vi "MeasInductance.vi"() -> ()   [LabVIEW 2017]
uses:
  <vilib>/Analysis/6fits.llb/Curve Fitting Criteria.ctl
  <vilib>/Analysis/NI_AALPro.lvlib
  Keysight N8731A conversion/Keysight N8900 Series.lvlib
panel:
  in  "filename":string caption="Discard data if empty"
  out "Resistance":dbl
  out "Inductance":dbl
  out "V(I)":T1(graph)
  out "Time Data":dbl[](array[numeric])
  out "Voltage Data":dbl[](array[numeric])
  out "Current Data":dbl[](array[numeric])
  out "I(t)":T1(graph)
  in  "stop":bool
  out "start time":dbl format="%_19f"
  in  "Measurement time [s]":dbl=240.0
  in  "OV Value (10V)":dbl=10.0
  in  "VISA resource name":refnum<visa-resource-name>
  in  "Keithley (1)/PSU (0)":bool=TRUE caption="Voltage Source"
  in  "Voltage limit [V]":dbl
  in  "Current limit [A]":dbl
  in  "Time between measurements [ms]":dbl
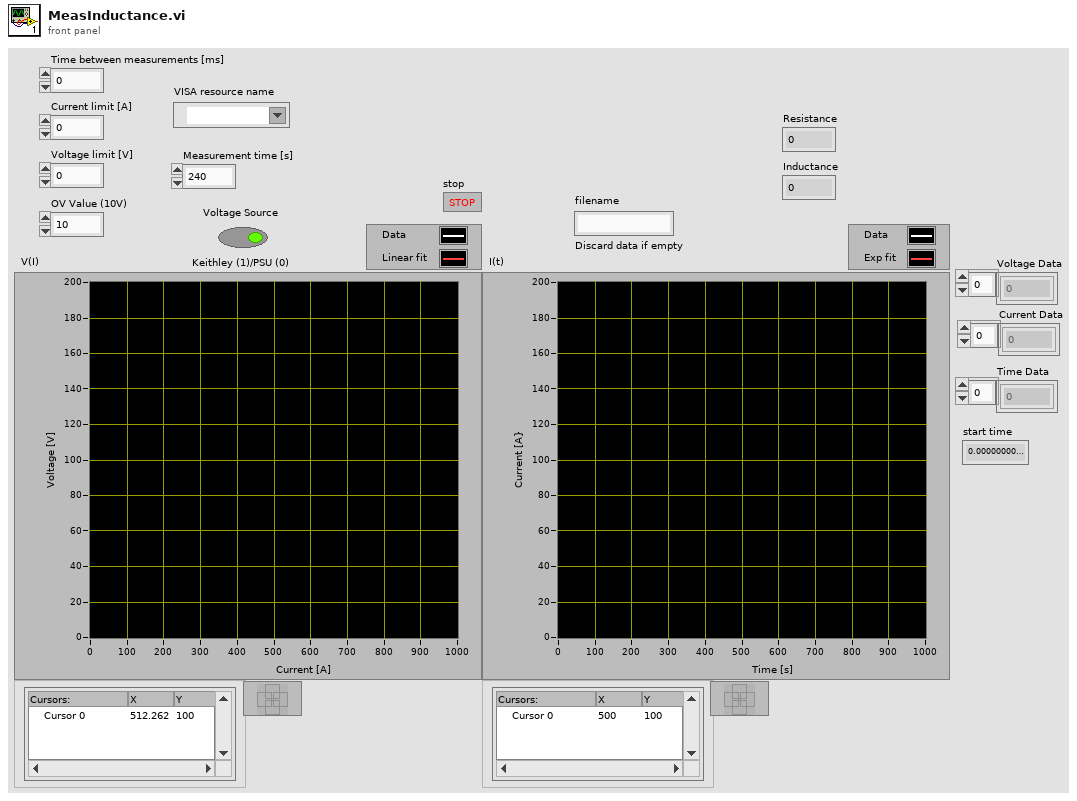
[diagram p1: front panel]
types:
  T1 = cluster{"Current Data":dbl[], "Best Linear Fit":dbl[]}[]
  T2 = cluster{"amp min":dbl, "amp max":dbl, "damping min":dbl, "damping max":dbl, "offset min":dbl, "offset max":dbl}
  T3 = typedef "NI_AALPro.lvlib/Curve Fitting Criteria.ctl" = u16
  T4 = cluster{"Current Data":dbl[], "Best Linear Fit":dbl[]}
  T5 = cluster{"Current Data":dbl[], "Voltage Data":dbl[]}
  T6 = cluster{"Time Data":dbl[], "Best Exponential Fit":dbl[]}
  T7 = cluster{"Time Data":dbl[], "Best Exponential Fit":dbl[]}[]
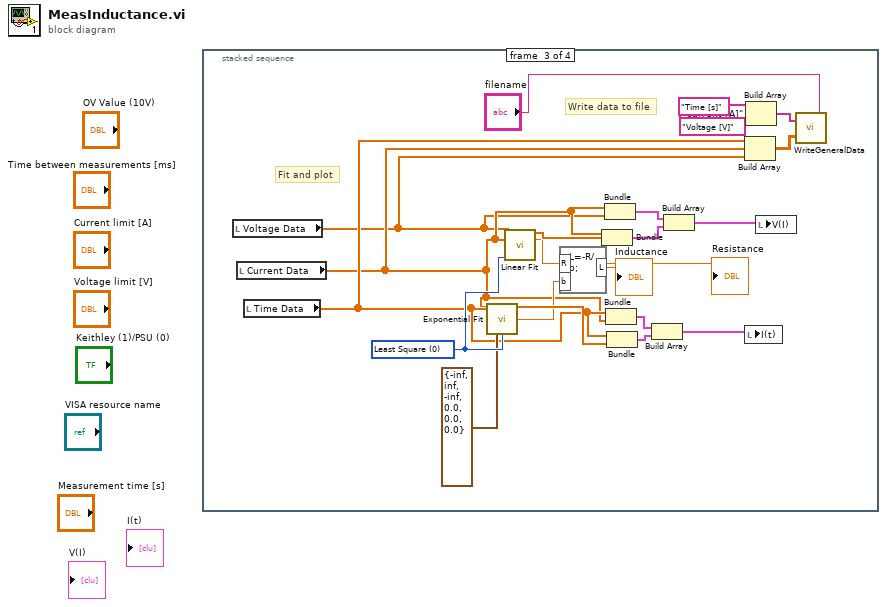
[diagram p0: block diagram]
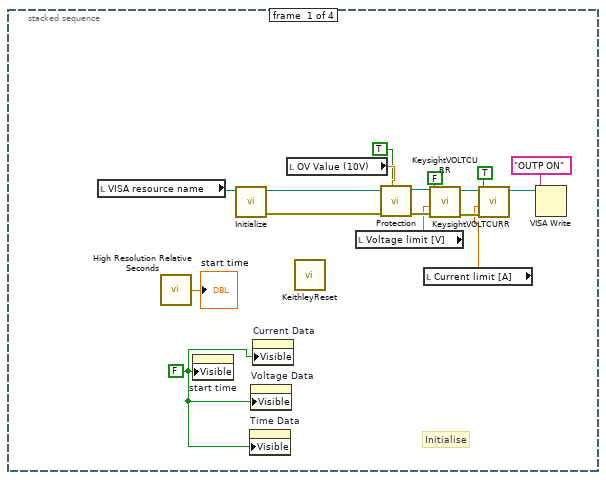
[diagram p2: hidden frame]
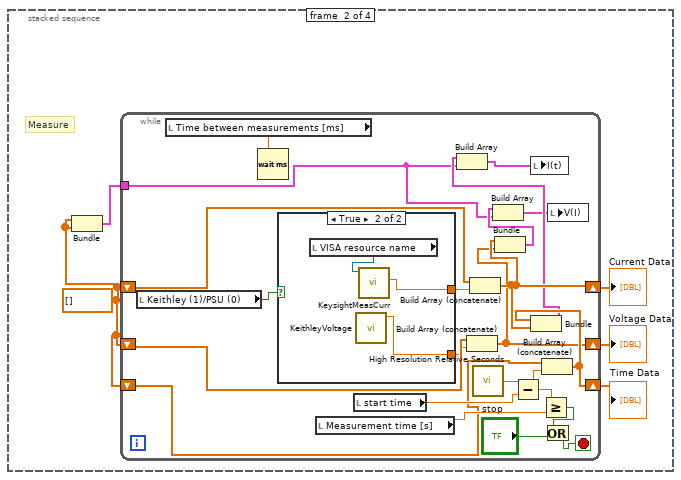
[diagram p3: hidden frame]
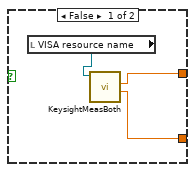
[diagram p4: hidden frame]
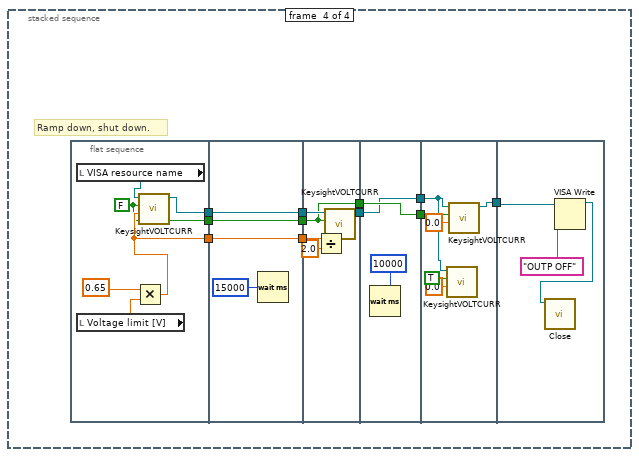
[diagram p5: hidden frame]
diagram:
  n1 = stacked-sequence {
    frame #0 {
      w3 = FALSE ("Visible")
      # "Initialise"
      n2 = local read "VISA resource name"() -> (w15:refnum<visa-resource-name>)
      n3 = call <vilib>:"High Resolution Relative Seconds.vi"() -> ("relative seconds"=→"start time":dbl)
      n4 = property on="start time" class="DigNum (strict)"("Visible"=w3) -> ()  [unwired: 2 in, 2 out]
      n5 = call "Initialize.vi"("VISA resource name"=w15) -> ("error out"=w17:errorcluster, "VISA resource name out"=w16:refnum<visa-resource-name>)  [unwired: 9 in]
      n6 = property on="Time Data" class="Arr (strict)"("Visible"=w3) -> ()  [unwired: 2 in, 2 out]
      n7 = property on="Voltage Data" class="Arr (strict)"("Visible"=w3) -> ()  [unwired: 2 in, 2 out]
      n8 = property on="Current Data" class="Arr (strict)"("Visible"=w3) -> ()  [unwired: 2 in, 2 out]
      n9 = local read "OV Value (10V)"() -> (w14:dbl)
      n10 = call "KeithleyReset.vi"() -> ()  [unwired: 11 in, 1 out]
      n11 = local read "Voltage limit [V]"() -> (w5:dbl)
      n12 = call "Protection.vi"("OV protection"=TRUE, "error in (no error)"=w17, "OV Value (10V)"=w14, "VISA resource name"=w16) -> ("error out"=w11:errorcluster, "VISA resource name out"=w12:refnum<visa-resource-name>)  [unwired: 6 in]
      n13 = local read "Current limit [A]"() -> (w6:dbl)
      n14 = call "KeysightVOLTCURR.vi"("error in (no error)"=w11, "CURR/VOLT (A/V)"=w5, "CURR (1)/VOLT (0)"=FALSE, "VISA resource name"=w12) -> ("error out"=w8:errorcluster, "VISA resource name out"=w9:refnum<visa-resource-name>)  [unwired: 6 in]
      n15 = call "KeysightVOLTCURR.vi"("error in (no error)"=w8, "CURR/VOLT (A/V)"=w6, "CURR (1)/VOLT (0)"=TRUE, "VISA resource name"=w9) -> ("VISA resource name out"=w2:refnum<visa-resource-name>)  [unwired: 6 in, 1 out]
      n16 = VISA Write(VISA resource name=w2, write buffer="OUTP ON") -> ()  [unwired: 1 in, 3 out]
    }
    frame #1 {
      w19 = dbl[] []
      # "Measure"
      n17 = Bundle(w19, w19) -> (w18:cluster{dbl[], dbl[]})  [unwired: 1 in]
      n18 = while {
        shift-right: [w29] -> w22
        shift-left: w19 -> [w41]
        shift-right: [w28] -> w21
        shift-left: w19 -> [w42]
        shift-right: [w30] -> w20
        shift-left: w19 -> [w31]
        tunnel: w18 -> [w25]
        stop <- w33 stop-if-true
        n19 = local read "Keithley (1)/PSU (0)"() -> (w43:bool)
        n20 = local read "Time between measurements [ms]"() -> (w44:dbl)
        n21 = Wait (ms)(milliseconds to wait=w44) -> ()  [unwired: 1 out]
        n22 = case shown="True" w43 {
          tunnel: [w46 w50] -> w40
          tunnel: [w45 w49] -> w39
          frame False {
            n23 = local read "VISA resource name"() -> (w47:refnum<visa-resource-name>)
            n24 = call "KeysightMeasBoth.vi"("VISA resource name"=w47) -> ("VOLT"=w45:dbl, "CURR"=w46:dbl)  [unwired: 7 in, 2 out]
          }
          frame True {
            n25 = local read "VISA resource name"() -> (w48:refnum<visa-resource-name>)
            n26 = call "KeithleyVoltage.vi"() -> ("Voltage"=w49:dbl)  [unwired: 10 in, 1 out]
            n27 = call "KeysightMeasCurr.vi"("VISA resource name"=w48) -> ("CURR"=w50:dbl)  [unwired: 8 in, 2 out]
          }
        }
        n28 = local read "Measurement time [s]"() -> (w36:dbl)
        n29 = local read "start time"() -> (w37:dbl)
        n30 = Build Array (concatenate)(w42, w39) -> (w28:dbl[])
        n31 = Build Array (concatenate)(w41, w40) -> (w29:dbl[])
        n32 = call <vilib>:"High Resolution Relative Seconds.vi"() -> ("relative seconds"=w38:dbl)
        n33 = Bundle(w29, w28) -> (w26:cluster{dbl[], dbl[]})  [unwired: 1 in]
        n34 = Build Array(w26, w25) -> (w23:cluster{dbl[], dbl[]}[])
        n35 = Subtract(x=w38, y=w37) -> (x-y=w32:dbl)
        n36 = Greater Or Equal?(x=w32, y=w36) -> (x >= y?=w35:bool)
        n37 = Build Array (concatenate)(w31, w32) -> (w30:dbl[])
        n38 = Bundle(w30, w29) -> (w27:cluster{dbl[], dbl[]})  [unwired: 1 in]
        n39 = Build Array(w27, w25) -> (w24:cluster{dbl[], dbl[]}[])
        n40 = local write "I(t)"(w24) -> ()
        n41 = Or(x=w35, y="stop") -> (x .or. y?=w33:bool)
        n42 = local write "V(I)"(w23) -> ()
      }
      "Current Data" <- w22
      "Voltage Data" <- w21
      "Time Data" <- w20
    }
    frame #2 {
      w72 = T3 0 items=["Least Square", "Least Absolute Residual", "Bisquare"] ("method")
      # "Write data to file"
      # "Fit and plot"
      n43 = local read "Voltage Data"() -> (w57:dbl[])
      n44 = local read "Current Data"() -> (w58:dbl[])
      n45 = local read "Time Data"() -> (w59:dbl[])
      n46 = call <vilib>:"Exponential Fit.vi"("Y"=w58, "X"=w59, "method"=w72, "parameter bounds"=T2 {"amp min"=-inf, "amp max"=inf, "damping min"=-inf, "damping max"=0.0, "offset min"=0.0, "offset max"=0.0}) -> ("Best Exponential Fit"=w66:dbl[], "damping"=w61:dbl)  [unwired: 6 in, 4 out]
      n47 = call <vilib>:"Linear Fit.vi"("Y"=w57, "X"=w58, "method"=w72) -> ("Best Linear Fit"=w71:dbl[], "slope"=w62:dbl)  [unwired: 8 in, 3 out]
      "Resistance" <- w62
      n48 = formula code="L=-R/b;"("b"=w61, "R"=w62) -> ("L"=→"Inductance":dbl)
      n49 = Bundle("Current Data"=w58, "Best Linear Fit"=w71) -> (w68:T4)  [unwired: 1 in]
      n50 = Bundle("Current Data"=w58, "Voltage Data"=w57) -> (w67:T5)  [unwired: 1 in]
      n51 = Bundle("Time Data"=w59, "Current Data"=w58) -> (w70:cluster{"Time Data":dbl[], "Current Data":dbl[]})  [unwired: 1 in]
      n52 = Bundle("Time Data"=w59, "Best Exponential Fit"=w66) -> (w69:T6)  [unwired: 1 in]
      n53 = Build Array(w70, w69) -> (w64:T7)
      n54 = Build Array(w67, w68) -> (w65:T1)
      n55 = Build Array(w59, w58, w57) -> (w52:dbl[][])
      n56 = local write "I(t)"(w64) -> ()
      n57 = Build Array("Time [s]", "Current [A]", "Voltage [V]") -> (w51:string[])
      n58 = local write "V(I)"(w65) -> ()
      n59 = call "WriteGeneralData.vi"("filename (discard if empty)"="filename", "Array"=w52, "Column name array"=w51) -> ()
    }
    frame #3 {
      # "Ramp down, shut down."
      n60 = flat-sequence {
        tunnel: [w86] -> w82
        tunnel: [w85] -> w80
        tunnel: [w84] -> w78
        tunnel: [w92] -> w83
        tunnel: w82 -> [w92]
        tunnel: [w91] -> w81
        tunnel: w80 -> [w91]
        tunnel: [w90] -> w79
        tunnel: w78 -> [w90]
        tunnel: w83 -> [w99]
        tunnel: w81 -> [w97]
        tunnel: w79 -> [w95]
        tunnel: [w95] -> w76
        tunnel: [w94] -> w74
        tunnel: [w101] -> w77
        tunnel: w76 -> [w101]
        tunnel: [w100] -> w75
        tunnel: w74 -> [w100]
        tunnel: w77 -> [w108]
        tunnel: w75 -> [w105]
        tunnel: [w103] -> w73
        tunnel: w73 -> [w111]
        frame #0 {
          w84 = FALSE ("CURR (1)/VOLT (0)")
          n61 = local read "VISA resource name"() -> (w89:refnum<visa-resource-name>)
          n62 = local read "Voltage limit [V]"() -> (w88:dbl)
          n63 = Multiply(x=0.65, y=w88) -> (x*y=w85:dbl)
          n64 = call "KeysightVOLTCURR.vi"("CURR/VOLT (A/V)"=w85, "CURR (1)/VOLT (0)"=w84, "VISA resource name"=w89) -> ("VISA resource name out"=w86:refnum<visa-resource-name>)  [unwired: 7 in, 1 out]
        }
        frame #1 {
          n65 = Wait (ms)(milliseconds to wait=u32 15000) -> ()  [unwired: 1 out]
        }
        frame #2 {
          n66 = Divide(x=w97, y=2.0) -> (x/y=w96:dbl)
          n67 = call "KeysightVOLTCURR.vi"("CURR/VOLT (A/V)"=w96, "CURR (1)/VOLT (0)"=w95, "VISA resource name"=w99) -> ("VISA resource name out"=w94:refnum<visa-resource-name>)  [unwired: 7 in, 1 out]
        }
        frame #3 {
          n68 = Wait (ms)(milliseconds to wait=u32 10000) -> ()  [unwired: 1 out]
        }
        frame #4 {
          n69 = call "KeysightVOLTCURR.vi"("CURR/VOLT (A/V)"=0.0, "CURR (1)/VOLT (0)"=TRUE, "VISA resource name"=w105) -> ()  [unwired: 7 in, 2 out]
          n70 = call "KeysightVOLTCURR.vi"("CURR/VOLT (A/V)"=0.0, "CURR (1)/VOLT (0)"=w108, "VISA resource name"=w105) -> ("VISA resource name out"=w103:refnum<visa-resource-name>)  [unwired: 7 in, 1 out]
        }
        frame #5 {
          n71 = VISA Write(VISA resource name=w111, write buffer="OUTP OFF") -> (VISA resource name out=w109:refnum<visa-resource-name>)  [unwired: 1 in, 2 out]
          n72 = call "Close.vi"("VISA resource name"=w109) -> ()  [unwired: 10 in, 1 out]
        }
      }
    }
  }
